vi "path.vi"(10 "Sample Name":string, 11 "Save Path & Template Directory":path) -> (3 "/Raw Data/":path)   [LabVIEW 2015]
panel:
  out "/<Sample Name>/":path
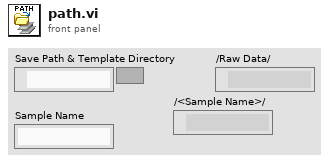
[diagram p1: front panel]
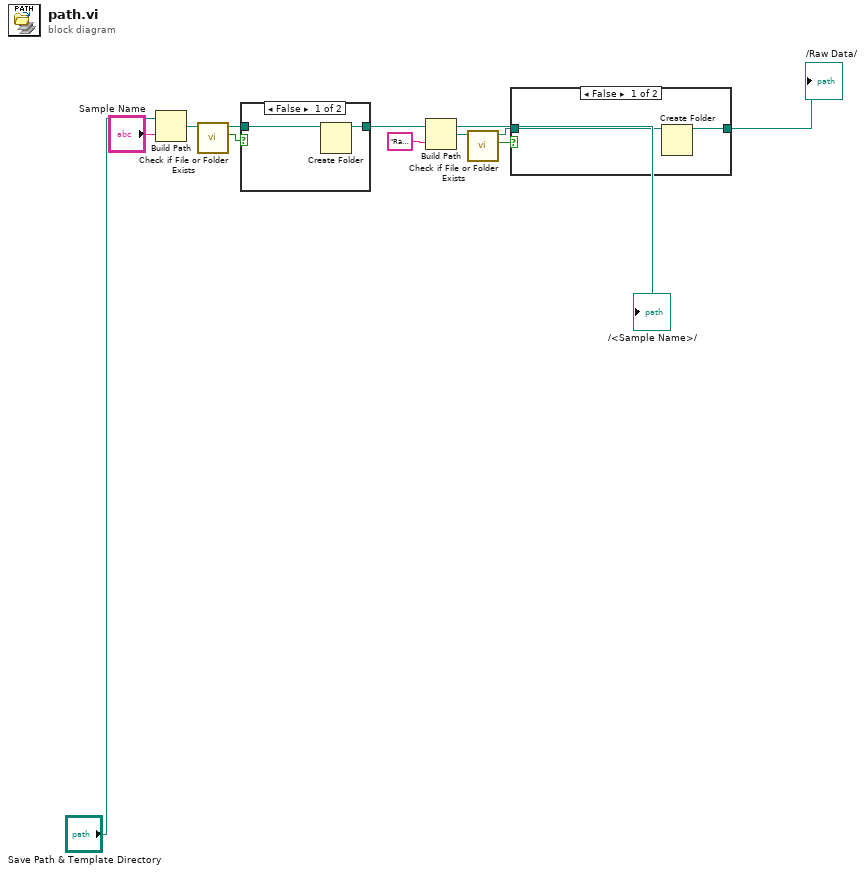
[diagram p0: block diagram]
diagram:
  n1 = Build Path(base path="Save Path & Template Directory", name or relative path="Sample Name") -> (appended path=w4:path)
  n2 = call <vilib>:"Check if File or Folder Exists.vi"("path"=w4) -> ("file or folder exists?"=w8:bool, "dup path"=w5:path)  [unwired: 8 in, 1 out]
  n3 = case shown="False" w8 {
    tunnel: [w13 w14] -> w10
    tunnel: w5 -> [w12 w14]
    frame False {
      n4 = Create Folder(path (use dialog)=w12) -> (created path=w13:path)  [unwired: 2 in, 2 out]
    }
    frame True {
    }
  }
  "/<Sample Name>/" <- w10
  n5 = Build Path(base path=w10, name or relative path="Raw Data" ("prompt (Create Folder)")) -> (appended path=w7:path)
  n6 = call <vilib>:"Check if File or Folder Exists.vi"("path"=w7) -> ("file or folder exists?"=w9:bool, "dup path"=w1:path)  [unwired: 8 in, 1 out]
  n7 = case shown="False" w9 {
    tunnel: w1 -> [w15 w17]
    tunnel: [w16 w17] -> w2
    frame False {
      n8 = Create Folder(path (use dialog)=w15) -> (created path=w16:path)  [unwired: 2 in, 2 out]
    }
    frame True {
    }
  }
  "/Raw Data/" <- w2
